vi "Cast State Callback VI.vi"(10 "error in (no error)":errorcluster, 11 "VI Refnum":refnum<vi>) -> (2 "error out":errorcluster, 3 "Casted Ref":refnum<vi>)   [LabVIEW 2020, in "Stream.lvlib" / "Endpoint.lvclass"]
uses:
  Endpoint.lvclass
  Connection/Connection.lvclass
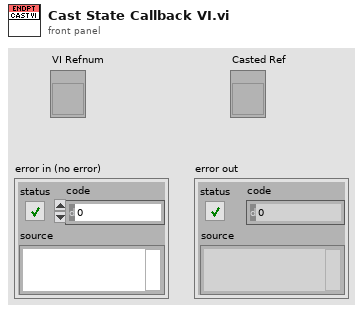
[diagram p1: front panel]
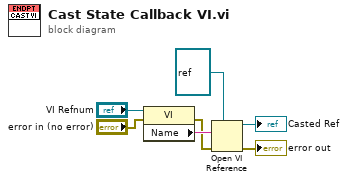
[diagram p0: block diagram]
diagram:
  n1 = property class="VI"(reference="VI Refnum", error in="error in (no error)") -> (error out=w1:errorcluster, "Name"=w5:string)  [unwired: 1 out]
  n2 = Open VI Reference(type specifier VI Refnum (for type only)=refnum<vi> refnum, vi path=w5, error in (no error)=w1) -> (vi reference=→"Casted Ref":refnum<vi>, error out=→"error out":errorcluster)  [unwired: 3 in]
